vi "Control_Rack_Controler.vi"(0 "Times":dbl[](array[numeric]), 1 "Voltages Toroidal (Keep below |10|)":dbl[](array[numeric]), 2 "Voltages Helical (Keep below |10|)":dbl[](array[numeric]), 3 "error out":errorcluster, 4 "Data out 2":T2) -> (5 "error out 2":errorcluster, 6 "Data out":T2)   [LabVIEW 2017]
uses:
  Type_Defs/Data.ctl
  Type_Defs/Diagnostics.ctl
  Type_Defs/Systems.ctl
  <vilib>/DAQmx/write.llb/DAQmx Write (Analog DBL 1Chan 1Samp).vi
  <vilib>/DAQmx/create/channels.llb/DAQmx Create Channel (AO-Voltage-Basic).vi
  <vilib>/DAQmx/miscellaneous.llb/DAQmx Fill In Error Info.vi
  <vilib>/express/express shared/transition.llb/Dynamic To Waveform Array.vi
  <vilib>/express/express signal manip/GetorSetDDTAttributes/Set DDT Attributes/SetT0.vi
  <vilib>/express/express shared/transition.llb/Waveform Array To Dynamic.vi
  <vilib>/express/express signal manip/GetorSetDDTAttributes/Set DDT Attributes/Set DDT Properties.xnode
panel:
  out "Toroidal Limited Current Set Point":dbl(graph)=-0.021820068359375
  out "Torroidal Voltage Feedback":dbl(graph)=-0.021820068359375
  out "Torroidal Current Feedback":dbl(graph)=-0.021820068359375
  out "Helix Current Feedback":dbl(graph)=-0.021820068359375
  out "Helix Voltage Feedback":dbl(graph)=-0.021820068359375
  out "Helix Limited Current Set Point":dbl(graph)=-0.021820068359375
  out "Experiment State":T1(ring)
  out "Experiment Purpose":string
  out "Start Time":timestamp
  out "Experiment Number":i32
  out "Operator":string
  out "Running":bool
  out "Voltage Toroidal":dbl
  out "Time":dbl
  out "Voltage Helical":dbl
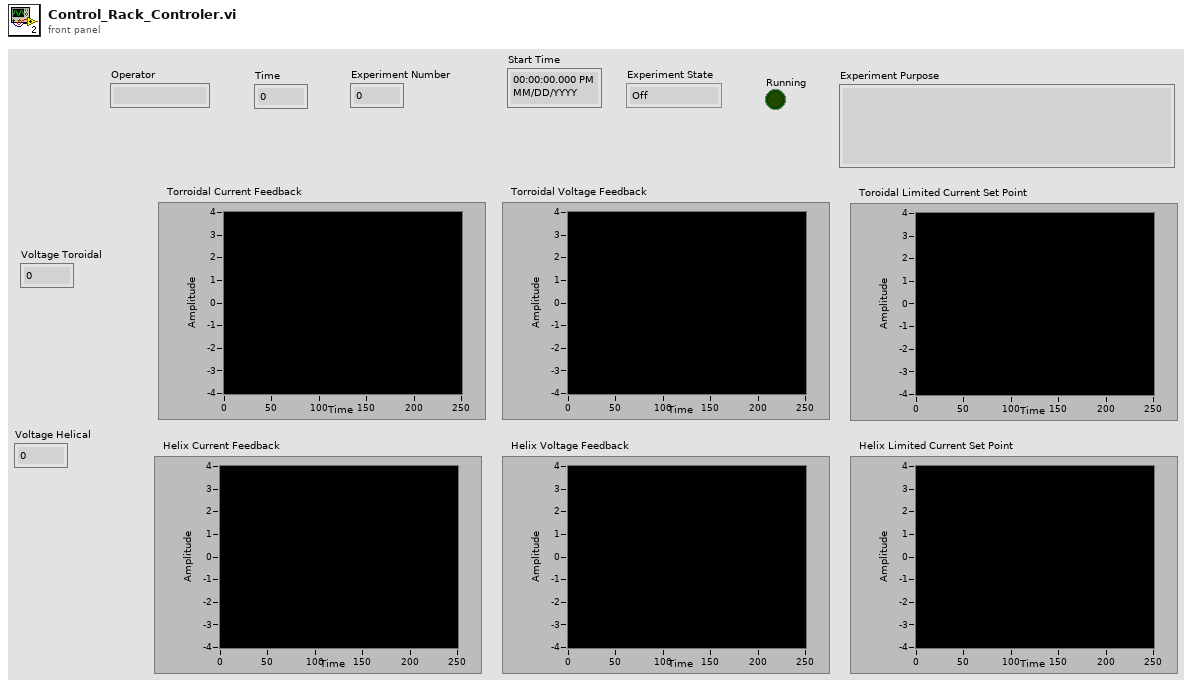
[diagram p1: front panel]
types:
  T1 = enum16{"Off", "Setting Up", "Ready", "In Progress", "Shutting Down"}
  T2 = typedef "Data.ctl" = cluster{"User Name":string, "Experiment Number":i32, "Start Time":timestamp, "Data":dbl[], "Step Number":i32, "Step Instructions":string, "Diagnostics":T3, "Experiment Purpose":string, "Experiment State":enum16{"Off", "Setting Up", "Ready", "In Progress", "Shutting Down"}, "Systems":T4, "Vacuum Pressure":dbl, "Fieldpoints":cluster{"System Boolean Fieldpoints":cluster{"Compressed Air":refnum<k21>, "T-20kV Power Switch":refnum<k21>, "T-Rectifier":refnum<k21>, "Engage Interlock":refnum<k21>, "Ventilator":refnum<k21>, "Magnetron":refnum<k21>, "H-20kV Power Switch":refnum<k21>, "H-Rectifier":refnum<k21>, "Main Water Pump":refnum<k21>, "WEGA Water Pump":refnum<k21>, "Gas Inlet Valves":refnum<k21>}, "Step Fieldpoints":cluster{"Exhaust Ventillator":refnum<k21>, "Compressed Air":refnum<k21>, "Water Pressure":refnum<k21>, "Interlock":refnum<k21>, "Toroidal Power Supply 1":refnum<k21>, "Toroidal Power Supply 2":refnum<k21>, "Toroidal Rectifier":refnum<k21>, "Helical Power Supply":refnum<k21>, "Helical Rectifier":refnum<k21>, "6kW Magnetron Standby":refnum<k21>, "20kW Magnetron Standby":refnum<k21>}}, "Pressure History":cluster{"Seconds into Experiment":i32[], "Pressure Data":dbl[]}, "Time Computer Control":dbl[], "Toroidal Voltage Computer Control":dbl[], "Helical Voltage Computer Control":dbl[], "Toroidal Current":dbl[], "Toroidal Voltage":dbl[], "Toroidal Current Set Point":dbl[], "Helical Current Set Point":dbl[], "Helical Voltage":dbl[], "Helical Current":dbl[], "Experiment Folder":path, "Run Another Shot?":bool}
  T3 = typedef "Diagnostics.ctl" = cluster{"Langmuir Probe":bool, "Rogowski 1":bool, "Rogowski 2":bool, "Rogowski 3":bool, "B-dot 1":bool, "B-dot 2":bool}
  T4 = typedef "Systems.ctl" = cluster{"Compressed Air":bool, "T-20kV Power Switch":bool, "T-Rectifier":bool, "Engage Interlock":bool, "Ventilator":bool, "Magnetron":bool, "H-20kV Power Switch":bool, "H-Rectifier":bool, "Main Water Pump":bool, "WEGA Water Pump":bool, "Gas Inlet Valves":bool}
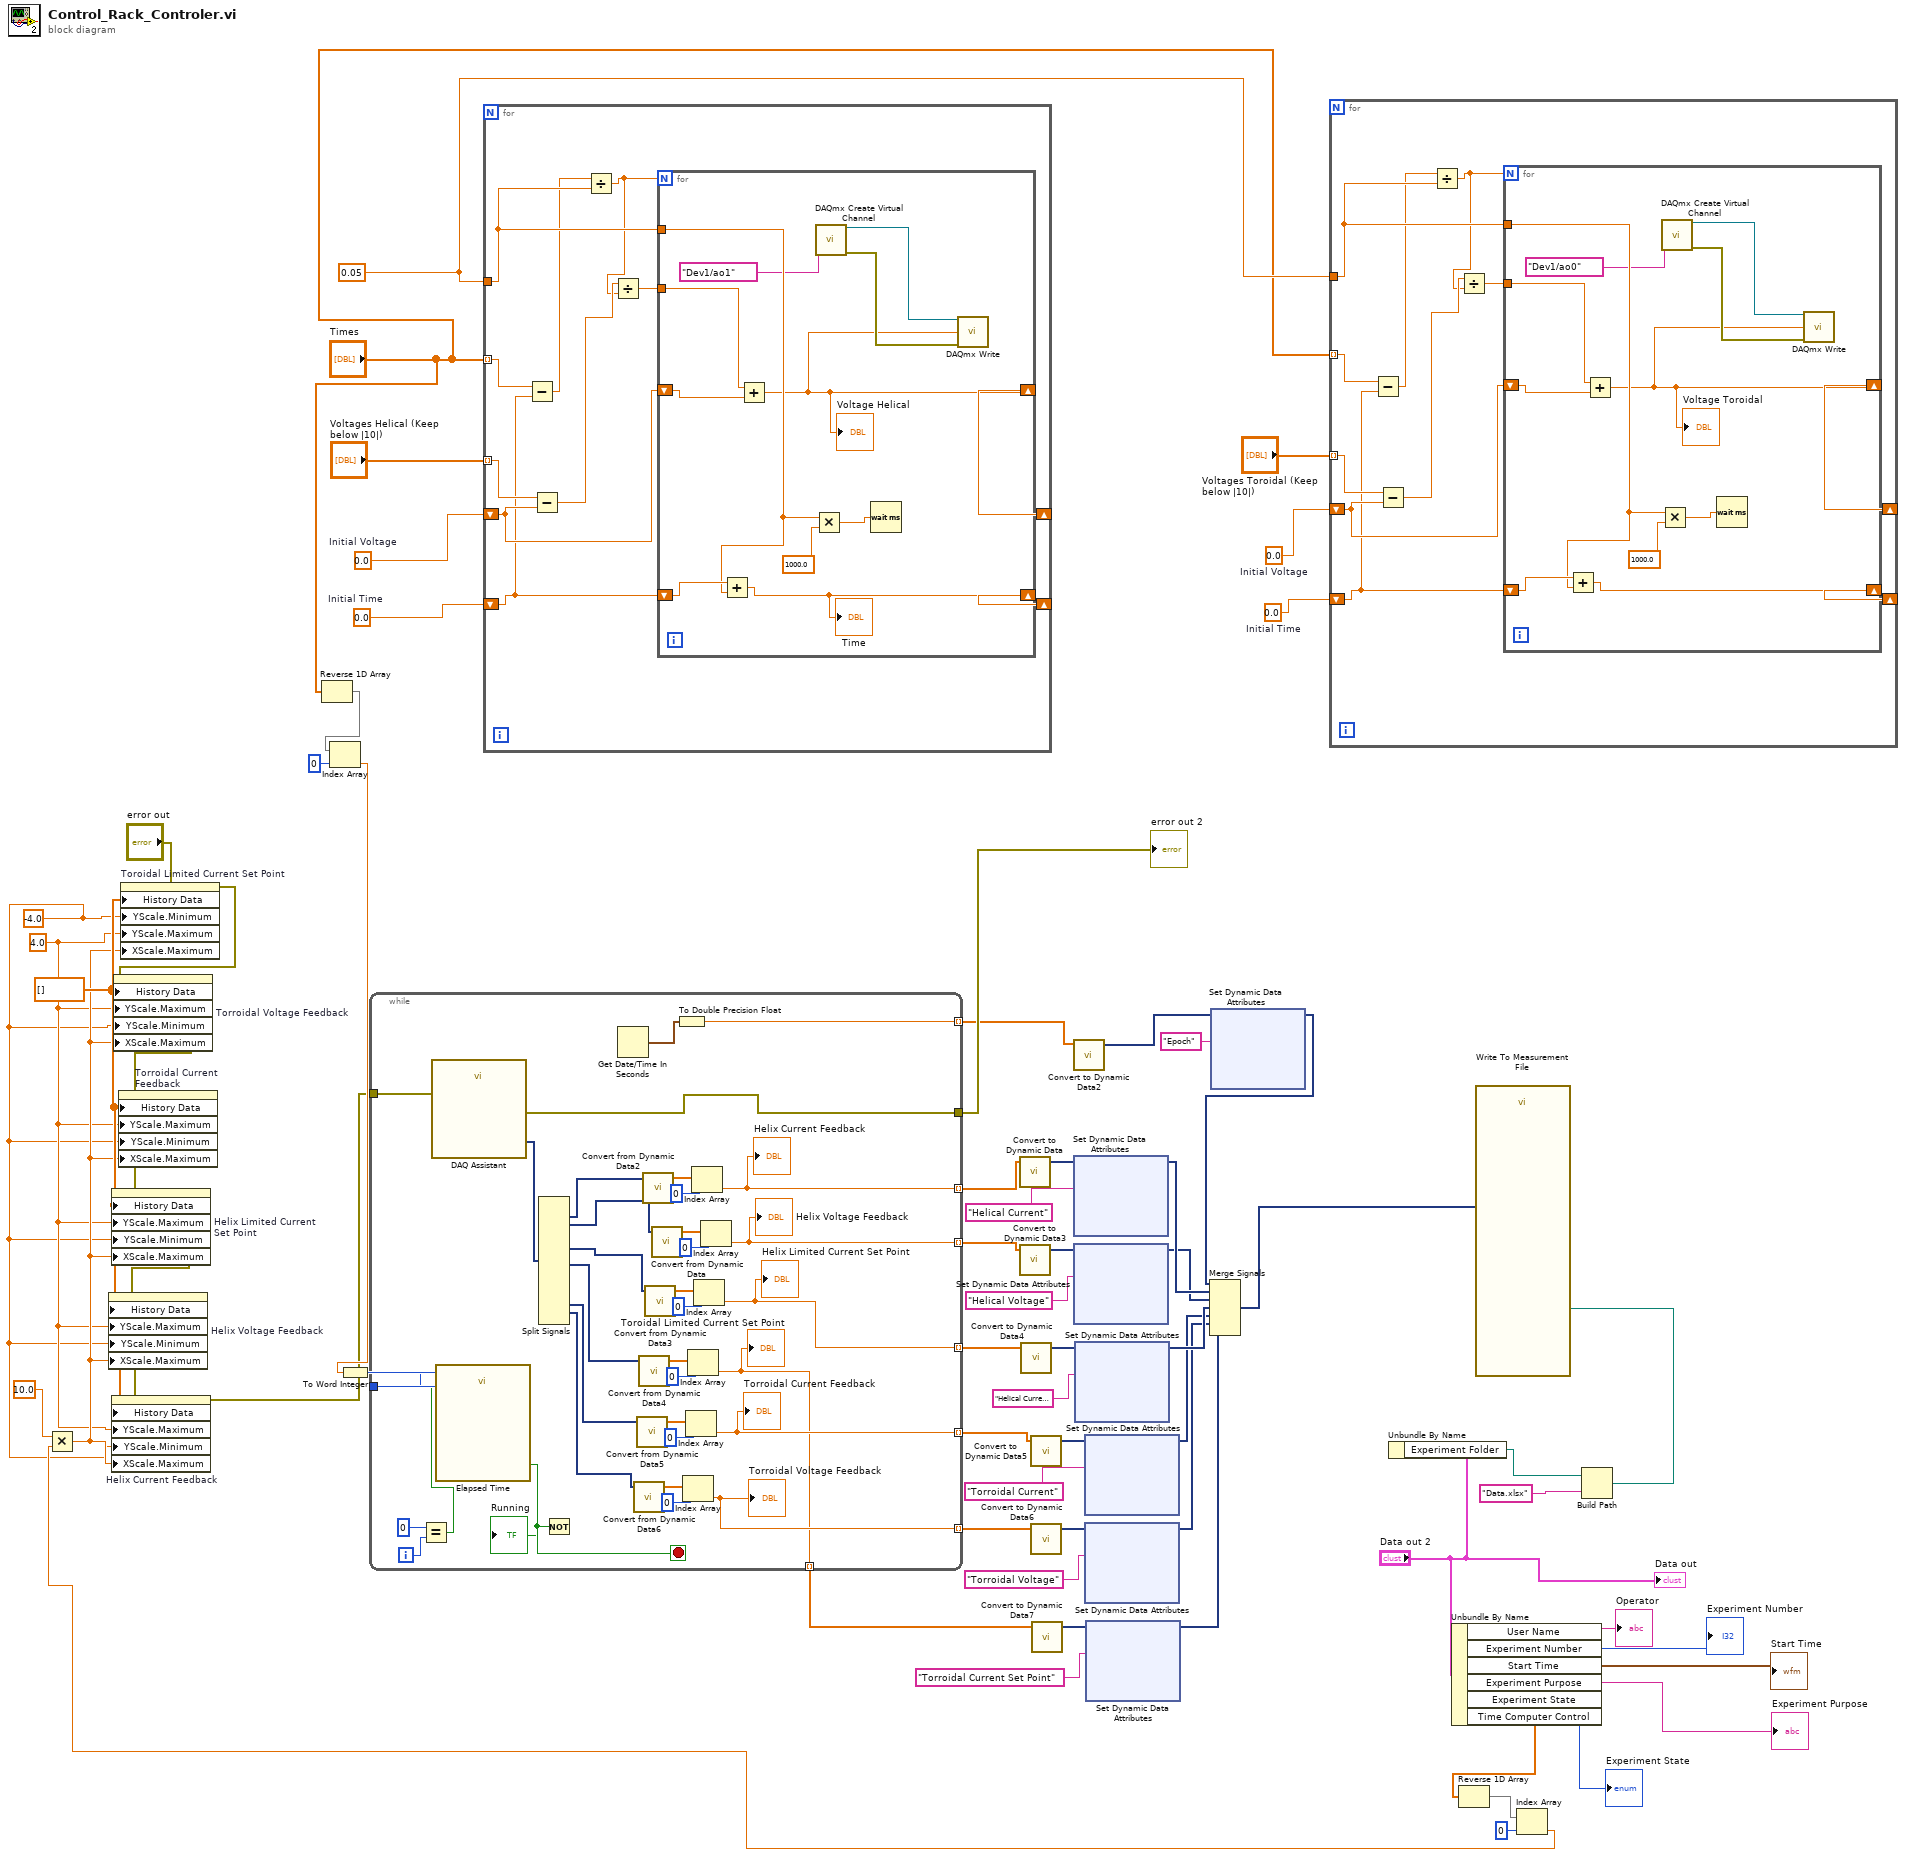
[diagram p0: block diagram]
diagram:
  w2 = 4.0 ("Y Scale.Range:Maximum")
  w1 = -4.0 ("Y Scale.Range:Minimum")
  w7 = dbl[] [] ("History Data")
  w61 = 0.05 ("Timestep (in seconds, keep above 1/20s)")
  w64 = 0.0  # Initial Time
  w63 = 0.0  # Initial Voltage
  w65 = 0.0  # Initial Time
  w66 = 0.0  # Initial Voltage
  n1 = Reverse 1D Array(array="Times") -> (reversed array=w59:dbl[])
  n2 = Index Array(array=w59, index=0) -> (element=w56:dbl)
  n3 = To Word Integer(number=w56) -> (16bit integer=w55:i16)
  n4 = for {
    tunnel: "Voltages Helical (Keep below |10|)" -> [w78] mode=indexing
    tunnel: "Times" -> [w71] mode=indexing
    tunnel: w61 -> [w73]
    shift-right: [w74] -> _
    shift-left: w66 -> [w77]
    shift-right: [w72] -> _
    shift-left: w65 -> [w70]
    n5 = Subtract(x=w71, y=w70) -> (x-y=w69:dbl)
    n6 = Subtract(x=w78, y=w77) -> (x-y=w76:dbl)
    n7 = Divide(x=w69, y=w73) -> (x/y=w68:dbl)
    n8 = Divide(x=w76, y=w68) -> (x/y=w75:dbl)
    n9 = for {
      N: w68 -> [_]
      shift-right: [w79] -> w74
      shift-left: w77 -> [w89]
      tunnel: w75 -> [w88]
      tunnel: w73 -> [w85]
      shift-right: [w83] -> w72
      shift-left: w70 -> [w87]
      n10 = Add(x=w87, y=w85) -> (x+y=w83:dbl)
      "Time" <- w83
      n11 = Add(x=w88, y=w89) -> (x+y=w79:dbl)
      "Voltage Helical" <- w79
      n12 = Multiply(x=w85, y=1000.0) -> (x*y=w86:dbl)
      n13 = call-poly <vilib>:"DAQmx Create Virtual Channel.vi"("physical channels"=tag "Dev1/ao1" ("write channel (torr = ao0, hel = ao1)")) -> ("task out"=w80:refnum<k21>, "error out"=w81:errorcluster)  [unwired: 13 in]
      n14 = Wait (ms)(milliseconds to wait=w86) -> ()  [unwired: 1 out]
      n15 = call-poly <vilib>:"DAQmx Write.vi"("task/channels in"=w80, "data"=w79, "error in"=w81) -> ()  [unwired: 10 in, 3 out]
    }
  }
  n16 = for {
    tunnel: "Voltages Toroidal (Keep below |10|)" -> [w100] mode=indexing
    tunnel: "Times" -> [w93] mode=indexing
    tunnel: w61 -> [w95]
    shift-right: [w96] -> _
    shift-left: w63 -> [w99]
    shift-right: [w94] -> _
    shift-left: w64 -> [w92]
    n17 = Subtract(x=w93, y=w92) -> (x-y=w91:dbl)
    n18 = Subtract(x=w100, y=w99) -> (x-y=w98:dbl)
    n19 = Divide(x=w91, y=w95) -> (x/y=w90:dbl)
    n20 = Divide(x=w98, y=w90) -> (x/y=w97:dbl)
    n21 = for {
      N: w90 -> [_]
      shift-right: [w101] -> w96
      shift-left: w99 -> [w111]
      tunnel: w97 -> [w110]
      tunnel: w95 -> [w107]
      shift-right: [w105] -> w94
      shift-left: w92 -> [w109]
      n22 = Add(x=w109, y=w107) -> (x+y=w105:dbl)
      n23 = Add(x=w110, y=w111) -> (x+y=w101:dbl)
      "Voltage Toroidal" <- w101
      n24 = Multiply(x=w107, y=1000.0) -> (x*y=w108:dbl)
      n25 = call-poly <vilib>:"DAQmx Create Virtual Channel.vi"("physical channels"=tag "Dev1/ao0" ("write channel (torr = ao0, hel = ao1) 2")) -> ("task out"=w102:refnum<k21>, "error out"=w103:errorcluster)  [unwired: 13 in]
      n26 = Wait (ms)(milliseconds to wait=w108) -> ()  [unwired: 1 out]
      n27 = call-poly <vilib>:"DAQmx Write.vi"("task/channels in"=w102, "data"=w101, "error in"=w103) -> ()  [unwired: 10 in, 3 out]
    }
  }
  n28 = Unbundle By Name("Data out 2") -> ("Experiment Folder"=w53:path)
  n29 = Unbundle By Name("Data out 2") -> ("User Name"=→"Operator":string, "Experiment Number"=→"Experiment Number":i32, "Start Time"=→"Start Time":timestamp, "Experiment Purpose"=→"Experiment Purpose":string, "Experiment State"=→"Experiment State":T1, "Time Computer Control"=w11:dbl[])
  n30 = Reverse 1D Array(array=w11) -> (reversed array=w10:dbl[])
  n31 = Index Array(array=w10, index=0) -> (element=w4:dbl)
  n32 = Multiply(x=10.0, y=w4) -> (x*y=w3:dbl)
  n33 = property on="Toroidal Limited Current Set Point" class="WFChart (strict)"(error in="error out", "History Data"=w7, "YScale.Minimum"=w1, "YScale.Maximum"=w2, "XScale.Maximum"=w3) -> (error out=w6:errorcluster)  [unwired: 1 in, 1 out]
  n34 = property on="Torroidal Voltage Feedback" class="WFChart (strict)"(error in=w6, "History Data"=w7, "YScale.Maximum"=w2, "YScale.Minimum"=w1, "XScale.Maximum"=w3) -> (error out=w16:errorcluster)  [unwired: 1 in, 1 out]
  n35 = property on="Torroidal Current Feedback" class="WFChart (strict)"(error in=w16, "History Data"=w7, "YScale.Maximum"=w2, "YScale.Minimum"=w1, "XScale.Maximum"=w3) -> (error out=w15:errorcluster)  [unwired: 1 in, 1 out]
  n36 = property on="Helix Limited Current Set Point" class="WFChart (strict)"(error in=w15, "History Data"=w7, "YScale.Maximum"=w2, "YScale.Minimum"=w1, "XScale.Maximum"=w3) -> (error out=w14:errorcluster)  [unwired: 1 in, 1 out]
  n37 = property on="Helix Voltage Feedback" class="WFChart (strict)"(error in=w14, "History Data"=w7, "YScale.Maximum"=w2, "YScale.Minimum"=w1, "XScale.Maximum"=w3) -> (error out=w13:errorcluster)  [unwired: 1 in, 1 out]
  n38 = property on="Helix Current Feedback" class="WFChart (strict)"(error in=w13, "History Data"=w7, "YScale.Maximum"=w2, "YScale.Minimum"=w1, "XScale.Maximum"=w3) -> (error out=w12:errorcluster)  [unwired: 1 in, 1 out]
  n39 = while {
    tunnel: [w119] -> w57
    tunnel: w55 -> [w145]
    tunnel: [w114] -> w19 mode=indexing
    tunnel: [w115] -> w30 mode=indexing
    tunnel: [w118] -> w29 mode=indexing
    tunnel: [w116] -> w28 mode=indexing
    tunnel: [w117] -> w27 mode=indexing
    tunnel: [w112] -> w26 mode=indexing
    tunnel: [w121] -> w18 mode=indexing
    tunnel: w12 -> [w113]
    i -> [w120]
    stop <- w124 stop-if-true
    n40 = Equal?(x=0, y=w120) -> (x = y?=w125:bool)
    n41 = call "DAQ Assistant"("error in"=w113) -> ("data"=w146:dynamicdata, "error out"=w119:errorcluster)  [unwired: 16 in, 1 out]
    n42 = call "Elapsed Time"("Time Target (s)"=w145, "Reset"=w125) -> ("Time has Elapsed"=w124:bool)  [unwired: 10 in, 7 out]
    n43 = Split Signals(w146) -> (w144:dynamicdata, w131:dynamicdata, w130:dynamicdata, w129:dynamicdata, w128:dynamicdata, w127:dynamicdata)  [unwired: 16 in, 10 out]
    n44 = Not(x=w124) -> (.not. x?=→"Running":bool)
    n45 = Get Date/Time In Seconds() -> (seconds since 1Jan1904=w122:timestamp)
    n46 = call "Convert from Dynamic Data6"("Dynamic Data Type"=w127) -> ("Array"=w133:dbl[])  [unwired: 3 in]
    n47 = call "Convert from Dynamic Data5"("Dynamic Data Type"=w128) -> ("Array"=w135:dbl[])  [unwired: 3 in]
    n48 = call "Convert from Dynamic Data4"("Dynamic Data Type"=w129) -> ("Array"=w137:dbl[])  [unwired: 3 in]
    n49 = call "Convert from Dynamic Data2"("Dynamic Data Type"=w144) -> ("Array"=w143:dbl[])  [unwired: 3 in]
    n50 = call "Convert from Dynamic Data3"("Dynamic Data Type"=w130) -> ("Array"=w139:dbl[])  [unwired: 3 in]
    n51 = call "Convert from Dynamic Data"("Dynamic Data Type"=w131) -> ("Array"=w141:dbl[])  [unwired: 3 in]
    n52 = To Double Precision Float(number=w122) -> (double precision float=w121:dbl)
    n53 = Index Array(array=w133, index=0) -> (element=w117:dbl)
    "Torroidal Voltage Feedback" <- w117
    n54 = Index Array(array=w135, index=0) -> (element=w116:dbl)
    "Torroidal Current Feedback" <- w116
    n55 = Index Array(array=w137, index=0) -> (element=w112:dbl)
    "Toroidal Limited Current Set Point" <- w112
    n56 = Index Array(array=w143, index=0) -> (element=w114:dbl)
    "Helix Current Feedback" <- w114
    n57 = Index Array(array=w139, index=0) -> (element=w118:dbl)
    "Helix Limited Current Set Point" <- w118
    n58 = Index Array(array=w141, index=0) -> (element=w115:dbl)
    "Helix Voltage Feedback" <- w115
  }
  "error out 2" <- w57
  n59 = call "Convert to Dynamic Data"("Array"=w19) -> ("Dynamic Data Type"=w51:dynamicdata)  [unwired: 3 in]
  n60 = call "Convert to Dynamic Data3"("Array"=w30) -> ("Dynamic Data Type"=w44:dynamicdata)  [unwired: 3 in]
  n61 = call "Convert to Dynamic Data4"("Array"=w29) -> ("Dynamic Data Type"=w43:dynamicdata)  [unwired: 3 in]
  n62 = call "Convert to Dynamic Data5"("Array"=w28) -> ("Dynamic Data Type"=w42:dynamicdata)  [unwired: 3 in]
  n63 = call "Convert to Dynamic Data6"("Array"=w27) -> ("Dynamic Data Type"=w40:dynamicdata)  [unwired: 3 in]
  n64 = call "Convert to Dynamic Data7"("Array"=w26) -> ("Dynamic Data Type"=w17:dynamicdata)  [unwired: 3 in]
  n65 = call "Convert to Dynamic Data2"("Array"=w18) -> ("Dynamic Data Type"=w49:dynamicdata)  [unwired: 3 in]
  n66 = xnode "Set Dynamic Data Attributes"("Signals In"=w51, "Signal Name"="Helical Current") -> ("Signals Out"=w47:dynamicdata)  [unwired: 2 in, 1 out]
  n67 = xnode "Set Dynamic Data Attributes"("Signals In"=w44, "Signal Name"="Helical Voltage") -> ("Signals Out"=w39:dynamicdata)  [unwired: 2 in, 1 out]
  n68 = xnode "Set Dynamic Data Attributes"("Signals In"=w43, "Signal Name"="Helical Current Set Point") -> ("Signals Out"=w38:dynamicdata)  [unwired: 2 in, 1 out]
  n69 = xnode "Set Dynamic Data Attributes"("Signals In"=w42, "Signal Name"="Torroidal Current") -> ("Signals Out"=w37:dynamicdata)  [unwired: 2 in, 1 out]
  n70 = xnode "Set Dynamic Data Attributes"("Signals In"=w40, "Signal Name"="Torroidal Voltage") -> ("Signals Out"=w36:dynamicdata)  [unwired: 2 in, 1 out]
  n71 = xnode "Set Dynamic Data Attributes"("Signals In"=w17, "Signal Name"="Torroidal Current Set Point") -> ("Signals Out"=w35:dynamicdata)  [unwired: 2 in, 1 out]
  n72 = xnode "Set Dynamic Data Attributes"("Signals In"=w49, "Signal Name"="Epoch") -> ("Signals Out"=w46:dynamicdata)  [unwired: 2 in, 1 out]
  n73 = Merge Signals(w46, w47, w39, w38, w37, w36, w35) -> (w45:dynamicdata)
  n74 = Build Path(base path=w53, name or relative path="Data.xlsx") -> (appended path=w54:path)
  n75 = call "Write To Measurement File"("Signals"=w45, "Filename"=w54) -> ()  [unwired: 15 in, 3 out]
  "Data out" <- "Data out 2"
